vi "纳清探头一键校准.vi"(4 "校准量程":u16, 5 "校准方式":u16, 6 "MB_Master输入":refnum<class "MB_Master.lvclass">, 7 "探头":T1(ring), 8 "error in (no error)":errorcluster caption="错误输入（无错误）", 9 "标液三":cluster{"标准值":sgl, "检测值":sgl, "原始值":sgl}, 10 "标液二":cluster{"标准值":sgl, "检测值":sgl, "原始值":sgl}, 11 "标液一":cluster{"标准值":sgl, "检测值":sgl, "原始值":sgl}) -> (0 "error out":errorcluster caption="错误输出")   [LabVIEW 2016, in "斯坦道多参数.lvlib"]
uses:
  <vilib>/Plasmionique/MB Master/MB_Master/MB_Master.lvclass
  <vilib>/Plasmionique/MB Master/MB Master.lvlib
panel:
  out "数组":u16[](array[numeric]) format="%04x"
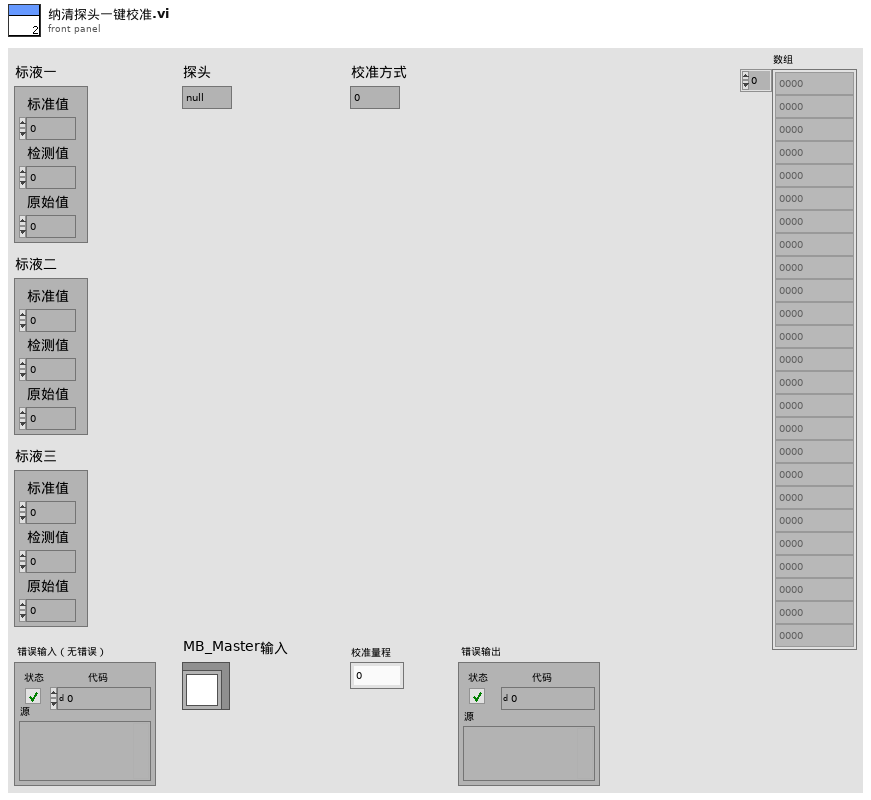
[diagram p1: front panel]
types:
  T1 = enum16{"null", "pH", "DO", "浊度", "电导率", "叶绿素a", "藻密度"}
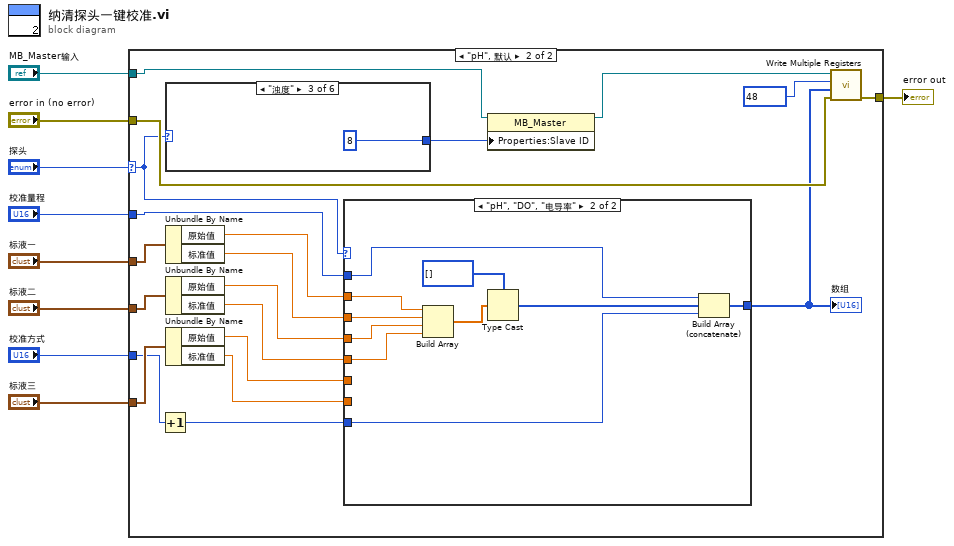
[diagram p0: block diagram]
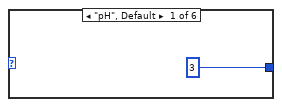
[diagram p3: hidden frame]
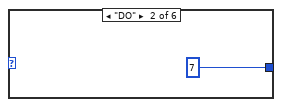
[diagram p4: hidden frame]
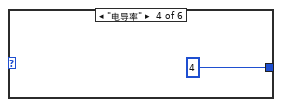
[diagram p5: hidden frame]
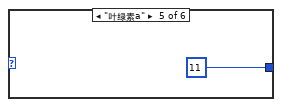
[diagram p6: hidden frame]
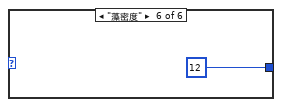
[diagram p7: hidden frame]
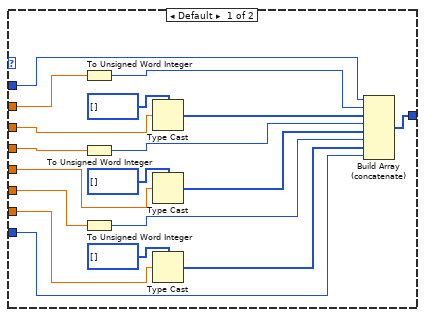
[diagram p8: hidden frame]
diagram:
  n1 = case shown="\"pH\", 默认" "探头" {
    selector: "探头" -> [_ w13]
    tunnel: "error in (no error)" -> [w10 w30]
    tunnel: [w10 w29] -> w8
    tunnel: "标液一" -> [_ w28]
    tunnel: "标液二" -> [_ w27]
    tunnel: "标液三" -> [_ w26]
    tunnel: "校准量程" -> [_ w19]
    tunnel: "校准方式" -> [_ w18]
    tunnel: "MB_Master输入" -> [_ w11]
    frame "null" {
    }
    frame "pH", Default {
      n2 = Increment(x=w18) -> (x+1=w17:u16)
      n3 = case shown="\"浊度\"" w13 {
        tunnel: [3 7 8 4 11 12] -> w16
        frame "pH", Default {
        }
        frame "DO" {
        }
        frame "浊度" {
        }
        frame "电导率" {
        }
        frame "叶绿素a" {
        }
        frame "藻密度" {
        }
      }
      n4 = Unbundle By Name(w28) -> ("原始值"=w25:sgl, "标准值"=w22:sgl)
      n5 = Unbundle By Name(w27) -> ("原始值"=w24:sgl, "标准值"=w21:sgl)
      n6 = Unbundle By Name(w26) -> ("原始值"=w23:sgl, "标准值"=w20:sgl)
      n7 = case shown="\"pH\", \"DO\", \"电导率\"" w13 {
        tunnel: w25 -> [w54 w63]
        tunnel: [w50 w57] -> w12
        tunnel: w24 -> [w49 w61]
        tunnel: w23 -> [w43 _]
        tunnel: w22 -> [w51 w62]
        tunnel: w21 -> [w47 w60]
        tunnel: w20 -> [w40 _]
        tunnel: w19 -> [w38 w56]
        tunnel: w17 -> [w37 w55]
        frame Default {
          n8 = To Unsigned Word Integer(number=w54) -> (unsigned 16bit integer=w53:u16)
          n9 = To Unsigned Word Integer(number=w49) -> (unsigned 16bit integer=w45:u16)
          n10 = To Unsigned Word Integer(number=w43) -> (unsigned 16bit integer=w42:u16)
          n11 = Type Cast(type=u16[] [], x=w51) -> (*(type *) &x=w46:u16[])
          n12 = Type Cast(type=u16[] [], x=w47) -> (*(type *) &x=w44:u16[])
          n13 = Type Cast(type=u16[] [], x=w40) -> (*(type *) &x=w39:u16[])
          n14 = Build Array (concatenate)(w38, w53, w46, w45, w44, w42, w39, w37) -> (w50:u16[])
        }
        frame "pH", "DO", "电导率" {
          n15 = Build Array(w63, w62, w61, w60) -> (w59:sgl[])
          n16 = Type Cast(type=u16[] [], x=w59) -> (*(type *) &x=w58:u16[])
          n17 = Build Array (concatenate)(w56, w58, w55) -> (w57:u16[])
        }
      }
      "数组" <- w12
      n18 = property class="MB_Master"(reference=w11, "Properties:Slave ID"=w16) -> (reference out=w15:refnum<class "MB_Master.lvclass">)  [unwired: 1 in, 1 out]
      n19 = call <vilib>:"Write Multiple Registers.vi"("error in (no error)"=w30, "values"=w12, "starting address"=u16 48, "MB session in"=w15) -> ("error out"=w29:errorcluster)  [unwired: 6 in, 1 out]
    }
  }
  "error out" <- w8
